vi "Read configuration.vi"(8 "error in":errorcluster, 11 "PLTarget CVS in":refnum<class "PLTarget CVS.lvclass">) -> (0 "error out":errorcluster, 2 "configuration":refnum<class "NISE_CEF_serializable configuration.lvclass">, 3 "PLTarget CVS out":refnum<class "PLTarget CVS.lvclass">)   [LabVIEW 2013, in "PLTarget CVS.lvclass"]
uses:
  PLTarget CVS.lvclass
  <vilib>/NI/Configuration Framework/serializable configuration/NISE_CEF_serializable configuration.lvclass
  PLTarget CVS.lvclass/PLTarget CVS.ctl
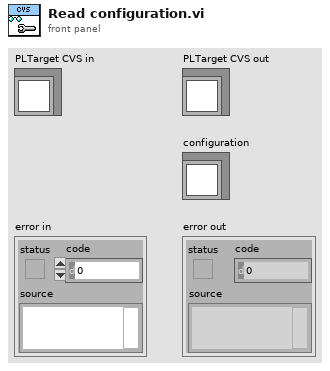
[diagram p1: front panel]
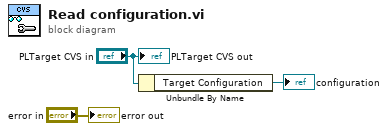
[diagram p0: block diagram]
diagram:
  n1 = Unbundle By Name("PLTarget CVS in") -> ("Target Configuration"=→"configuration":refnum<class "PL_Target Configuration.lvclass">)
  "error out" <- "error in"
  "PLTarget CVS out" <- "PLTarget CVS in"
